vi "MAC_HexToColon.vi"(11 "MAC Address (hex string)":string) -> (3 "MAC Address (colon notation)":string)   [LabVIEW 2022 SP3, in "hse-network.lvlib"]
doc: "(v0.2.1b; 2017-08-14 16:44)\n\n\n\n____\nHAMPEL SOFTWARE ENGINEERING v3.8.0 (2023-12-18 14:41)"
uses:
  hse-network.lvlib
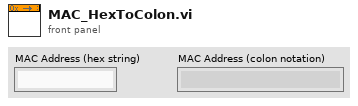
[diagram p1: front panel]
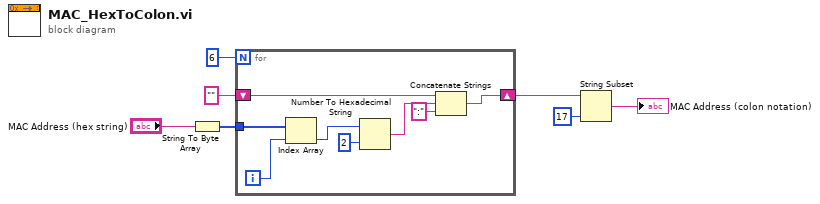
[diagram p0: block diagram]
diagram:
  n1 = String To Byte Array(string="MAC Address (hex string)") -> (unsigned byte array=w6:u8[])
  n2 = for {
    N: 6 -> [_]
    tunnel: w6 -> [w10]
    shift-right: [w12] -> w3
    shift-left: "" -> [w14]
    i -> [w9]
    n3 = Index Array(array=w10, index=w9) -> (element=w8:u8)
    n4 = Number To Hexadecimal String(1:i16 2 ("width (-)"), 2:w8) -> (0:w13:string)
    n5 = Concatenate Strings(w14, w13, ":" ("string")) -> (w12:string)
  }
  n6 = String Subset(string=w3, length (rest)=17 ("length (rest)")) -> (substring=→"MAC Address (colon notation)":string)  [unwired: 1 in]
